vi "NanoScan Send Command.vi"(0 "VISA Ref":refnum<visa-resource-name>, 2 "Wait for Reply (T)":bool=TRUE, 7 "Command":string, 11 "Error In":errorcluster) -> (4 "VISA Ref Dup":refnum<visa-resource-name>, 8 "Reply":string, 13 "Cmd Success":bool, 15 "Error Out":errorcluster)   [LabVIEW 2020]
uses:
  <vilib>/Utility/error.llb/whitespace.ctl
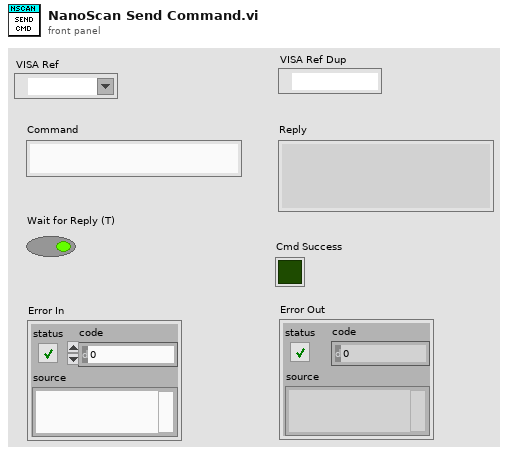
[diagram p1: front panel]
types:
  T1 = typedef "whitespace.ctl" = u16
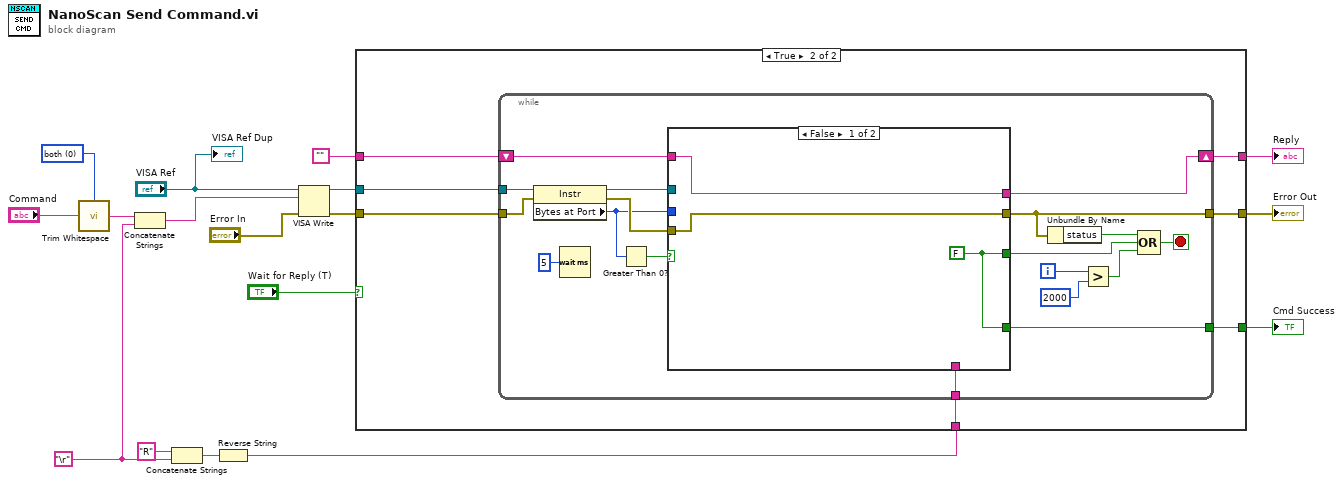
[diagram p0: block diagram]
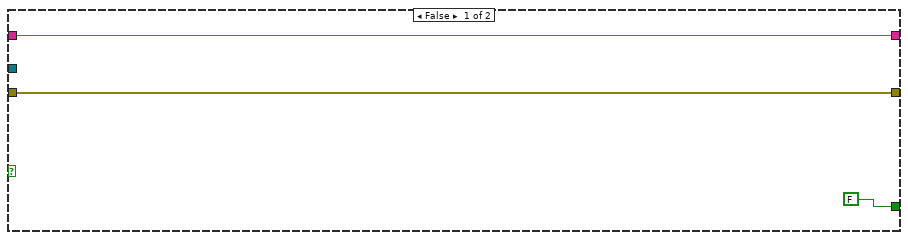
[diagram p2: hidden frame]
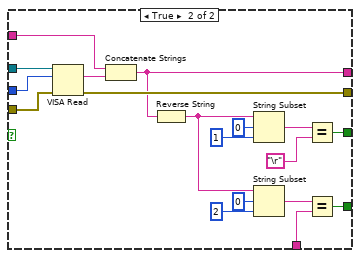
[diagram p3: hidden frame]
diagram:
  w4 = "\r"
  w16 = T1 0 items=["both", "start of string", "end of string"] ("location (both)")
  n1 = call <vilib>:"Trim Whitespace.vi"("string"="Command", "location (both)"=w16) -> ("trimmed string"=w15:string)
  n2 = Concatenate Strings(w15, w4) -> (w14:string)
  n3 = Concatenate Strings("R" ("string"), w4) -> (w2:string)
  n4 = Reverse String(1:w2) -> (0:w1:string)
  n5 = VISA Write(VISA resource name="VISA Ref", write buffer=w14, error in (no error)="Error In") -> (VISA resource name out=w13:refnum<visa-resource-name>, error out=w12:errorcluster)  [unwired: 1 out]
  n6 = case shown="True" "Wait for Reply (T)" {
    tunnel: w13 -> [_ w24]
    tunnel: w12 -> [w20 w23]
    tunnel: "" -> [w19 w27]
    tunnel: [w19 w26] -> w6
    tunnel: [w20 w25] -> w8
    tunnel: [FALSE w22] -> w5
    tunnel: w1 -> [_ w21]
    frame False {
    }
    frame True {
      n7 = while {
        tunnel: w24 -> [w45]
        tunnel: w23 -> [w44]
        shift-right: [w33] -> w26
        shift-left: w27 -> [w34]
        tunnel: [w31] -> w25
        tunnel: [w28] -> w22
        tunnel: w21 -> [w29]
        i -> [w43]
        stop <- w40 stop-if-true
        n8 = property class="Instr"(reference=w45, error in=w44) -> (reference out=w36:refnum<visa-resource-name>, error out=w37:errorcluster, "Bytes at Port"=w35:u32)
        n9 = Wait (ms)(milliseconds to wait=u32 5) -> ()  [unwired: 1 out]
        n10 = Greater Than 0?(x=w35) -> (x > 0?=w38:bool)
        n11 = case shown="False" w38 {
          tunnel: w37 -> [w48 w65]
          tunnel: w36 -> [_ w66]
          tunnel: w35 -> [_ w64]
          tunnel: w34 -> [w47 w63]
          tunnel: [w47 w60] -> w33
          tunnel: [w48 w61] -> w31
          tunnel: [w46 w56] -> w30
          tunnel: w29 -> [_ w50]
          tunnel: [w46 w49] -> w28
          frame False {
            w46 = FALSE
          }
          frame True {
            n12 = VISA Read(VISA resource name=w66, byte count=w64, error in (no error)=w65) -> (read buffer=w62:string, error out=w61:errorcluster)  [unwired: 2 out]
            n13 = Concatenate Strings(w63, w62) -> (w60:string)
            n14 = Reverse String(1:w60) -> (0:w54:string)
            n15 = String Subset(string=w54, offset (0)=0, length (rest)=1 ("length (rest)")) -> (substring=w57:string)
            n16 = String Subset(string=w54, offset (0)=0, length (rest)=2 ("length (rest)")) -> (substring=w51:string)
            n17 = Equal?(x=w57, y="\r") -> (x = y?=w56:bool)
            n18 = Equal?(x=w51, y=w50) -> (x = y?=w49:bool)
          }
        }
        n19 = Unbundle By Name(w31) -> ("status"=w32:bool)
        n20 = Greater?(x=w43, y=2000) -> (0:w41:bool)
        n21 = Compound Arithmetic op=OR(w32, w30, w41) -> (w40:bool)
      }
    }
  }
  "Reply" <- w6
  "Error Out" <- w8
  "Cmd Success" <- w5
  "VISA Ref Dup" <- "VISA Ref"
